vi "SMU.SetOutput.vi"(8 "error in (no error)":errorcluster, 10 "Output (False)":bool, 11 "SMU.Keithley2600 in":refnum<class "SMU.Keithley2600.lvclass">) -> (0 "error out":errorcluster, 3 "SMU.Keithley2600 out":refnum<class "SMU.Keithley2600.lvclass">)   [LabVIEW 2019, in "SMU.Keithley2600.lvclass"]
uses:
  SMU.Keithley2600.lvclass
  <instrlib>/Keithley 2600 Series/Keithley 2600 Series.lvlib
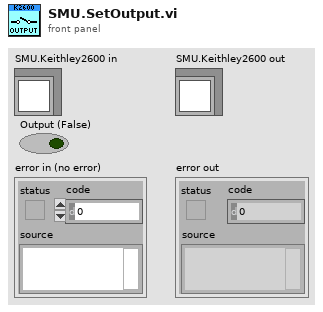
[diagram p1: front panel]
types:
  T1 = typedef "SMU.Keithley2600.lvclass/Resource--Cluster.ctl" = cluster{"VISA resource":refnum<visa-resource-name>, "Channel":i32}
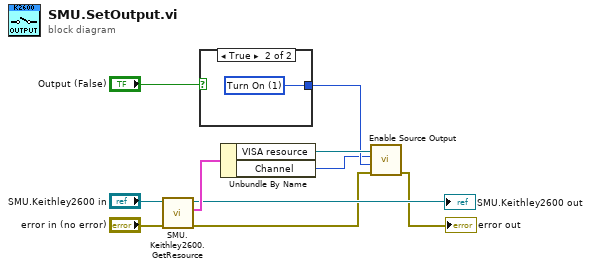
[diagram p0: block diagram]
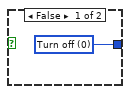
[diagram p2: hidden frame]
diagram:
  n1 = call "SMU.Keithley2600.GetResource.vi"("error in (no error)"="error in (no error)", "SMU.Keithley2600 in"="SMU.Keithley2600 in") -> ("error out"=w2:errorcluster, "Resource"=w8:T1, "SMU.Keithley2600 out"=→"SMU.Keithley2600 out":refnum<class "SMU.Keithley2600.lvclass">)  [unwired: 7 in]
  n2 = case shown="True" "Output (False)" {
    tunnel: [w11 w12] -> w4
    frame False {
      w11 = 0 items=["Turn off", "Turn On", "High-Z"] ("Output Mode (0: Turn off)")
    }
    frame True {
      w12 = 1 items=["Turn off", "Turn On", "High-Z"] ("Output Mode (0: Turn off)")
    }
  }
  n3 = Unbundle By Name(w8) -> ("VISA resource"=w6:refnum<visa-resource-name>, "Channel"=w3:i32)
  n4 = call <instrlib>:"Enable Source Output.vi"("error in (no error)"=w2, "Output Mode (0: Turn off)"=w4, "Source Measure Unit Channel (0: Channel A)"=w3, "VISA resource name"=w6) -> ("error out"=→"error out":errorcluster)  [unwired: 6 in, 1 out]
